vi "Flatten U64.vi"(3 "U64":u64, 4 "Endian":T1) -> (5 "Flat Data":u8[](array[numeric]) format="%.0x")   [LabVIEW 2021, in "DataTypes_CIF_U.lvlib"]
uses:
  DataTypes_CIF_U.lvlib
  Typedef/Endian.ctl
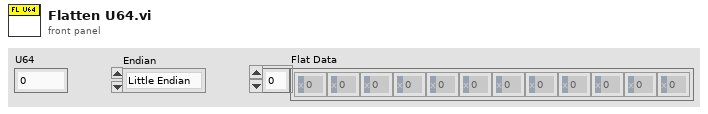
[diagram p1: front panel]
types:
  T1 = typedef "DataTypes_CIF_U.lvlib/Endian.ctl" = enum16{"Little Endian", "Big Endian"}
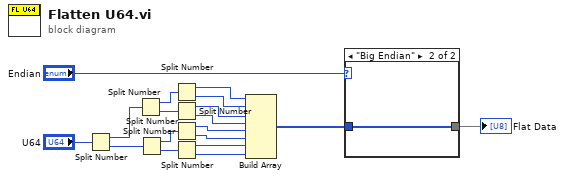
[diagram p0: block diagram]
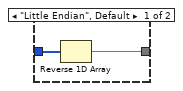
[diagram p2: hidden frame]
diagram:
  n1 = Split Number(x="U64") -> (hi(x)=w7:u32, lo(x)=w8:u32)
  n2 = Split Number(x=w7) -> (hi(x)=w5:u16, lo(x)=w6:u16)
  n3 = Split Number(x=w8) -> (hi(x)=w10:u16, lo(x)=w14:u16)
  n4 = Split Number(x=w5) -> (hi(x)=w1:u8, lo(x)=w2:u8)
  n5 = Split Number(x=w6) -> (hi(x)=w3:u8, lo(x)=w4:u8)
  n6 = Split Number(x=w10) -> (hi(x)=w11:u8, lo(x)=w12:u8)
  n7 = Split Number(x=w14) -> (hi(x)=w13:u8, lo(x)=w15:u8)
  n8 = Build Array(w1, w2, w3, w4, w11, w12, w13, w15) -> (w18:u8[])
  n9 = case shown="\"Big Endian\"" "Endian" {
    tunnel: w18 -> [w20 w21]
    tunnel: [w19 w21] -> w16
    frame "Little Endian", Default {
      n10 = Reverse 1D Array(array=w20) -> (reversed array=w19:u8[])
    }
    frame "Big Endian" {
    }
  }
  "Flat Data" <- w16
